vi "ConfigureMcsaAcquisition.vi"(8 "error in (no error)":errorcluster) -> (0 "error out":errorcluster, 2 "register data sets":T1[](array[typedef]), 3 "Mcsa Acquisition Config":T4 {"FixedSizeX31"."InputConfig" items=["AC Coupled", "DC Coupled", "IEPE AC Coupled"]}, 5 "valid":bool)   [LabVIEW 2017, in "McsaFpgaAcquisition.lvlib"]
uses:
  <vilib>/addons/InsightCM/Devices/Shared/Mcsa/McsaFpgaAcquisition/McsaFpgaAcquisition.lvlib
  <vilib>/addons/InsightCM/Devices/Shared/Mcsa/McsaFpgaAcquisition/controls/Configuration.ctl
  <vilib>/addons/InsightCM/Devices/Shared/Cms/CmsAcquisition/controls/FixedSizeArrays.ctl
  <vilib>/LabVIEW Targets/FPGA/cRIO/shared/nicrio_ModuleControls/nicrio_cRIO-9232_ConfigModeRing.ctl
  <vilib>/addons/InsightCM/Devices/Shared/Cms/cRIOWfmAcq/subVIs/RIO Wfm Cust Ctrls/rwfm_SamplingInfo.ctl
  <vilib>/addons/InsightCM/Devices/Shared/Mcsa/McsaFpgaAcquisition/controls/Group.ctl
  <vilib>/addons/InsightCM/Devices/Shared/Mcsa/McsaFpgaAcquisition/controls/ChannelMcsa.ctl
  <vilib>/addons/InsightCM/Devices/Shared/Mcsa/McsaFpgaAcquisition/controls/RangeParams.ctl
  <vilib>/addons/InsightCM/Devices/Shared/Mcsa/McsaDataEventCreator/controls/RegisterDataSets.ctl
  <vilib>/addons/InsightCM/Devices/Shared/Mcsa/McsaDataEventCreator/controls/Registry_DataSet.ctl
  <vilib>/addons/InsightCM/Devices/Shared/Mcsa/McsaDataEventCreator/controls/DataSetType.ctl
  <vilib>/addons/InsightCM/Utilities/GlobalConfiguration/GlobalConfiguration.lvlib
  <vilib>/addons/InsightCM/Devices/Shared/Cms/cRIOWfmAcq/cRIOWfmLib.lvlib
  <vilib>/addons/InsightCM/Devices/Shared/Cms/CmsAcquisition/CmsAcquisition.lvlib
  <vilib>/addons/InsightCM/Devices/Shared/Mcsa/McsaDataEventCreator/McsaDataEventCreator.lvlib
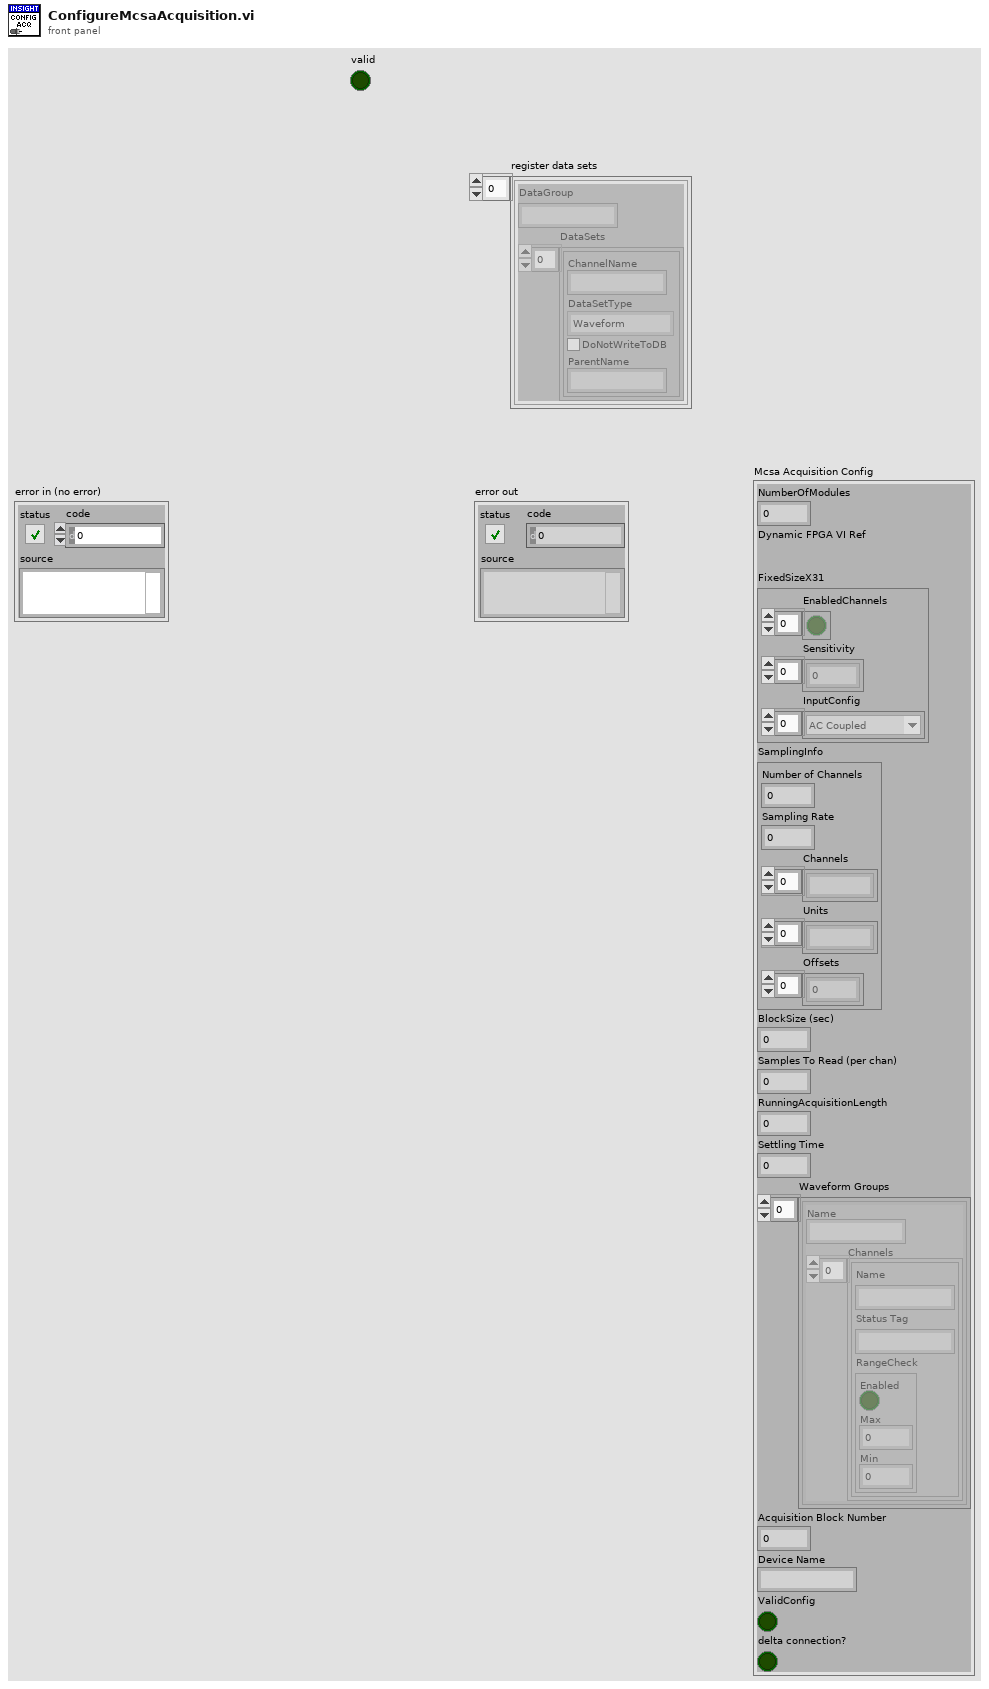
[diagram p1: front panel]
types:
  T1 = typedef "McsaDataEventCreator.lvlib/RegisterDataSets.ctl" = cluster{"DataGroup":string, "DataSets":T2[]}
  T2 = typedef "McsaDataEventCreator.lvlib/Registry_DataSet.ctl" = cluster{"ChannelName":string, "DataSetType":T3, "DoNotWriteToDB":bool, "ParentName":string}
  T3 = typedef "McsaDataEventCreator.lvlib/DataSetType.ctl" = enum16{"Waveform", "MCSAFFT", "TorqueWFM"}
  T4 = typedef "McsaFpgaAcquisition.lvlib/Configuration.ctl" = cluster{"NumberOfModules":i16, "Dynamic FPGA VI Ref":refnum<k20>, "FixedSizeX31":T5, "SamplingInfo":T7, "BlockSize (sec)":dbl, "Samples To Read (per chan)":i32, "RunningAcquisitionLength":dbl, "Settling Time":dbl, "Waveform Groups":T8[], "Acquisition Block Number":i32, "Device Name":string, "ValidConfig":bool, "delta connection?":bool}
  T5 = typedef "CmsAcquisition.lvlib/FixedSizeArrays.ctl" = cluster{"EnabledChannels":bool[], "Sensitivity":dbl[], "InputConfig":T6[]}
  T6 = typedef "nicrio_cRIO-9232_ConfigModeRing.ctl" = u8
  T7 = typedef "cRIOWfmLib.lvlib/rwfm_SamplingInfo.ctl" = cluster{"Number of Channels":i32, "Sampling Rate":dbl, "Channels":string[], "Units":string[], "Offsets":sgl[]}
  T8 = typedef "McsaFpgaAcquisition.lvlib/Group.ctl" = cluster{"Name":string, "Channels":T9[]}
  T9 = typedef "McsaFpgaAcquisition.lvlib/ChannelMcsa.ctl" = cluster{"Name":string, "Status Tag":string, "RangeCheck":T10}
  T10 = typedef "McsaFpgaAcquisition.lvlib/RangeParams.ctl" = cluster{"Enabled":bool, "Max":dbl, "Min":dbl}
  T11 = typedef "R2_Device.ctl" = cluster{"Id":string, "Name":string, "DeviceType":string, "HardwareName":string, "IpAddress":string, "HardwareInfo":T12[], "ApplicationType":string, "ApplicationVersion":string, "EquipmentIds":string[], "ConfigurationVersion":string, "State":T13, "Properties":T12[], "DataGroups":T14[], "BurstModeTrigger":T18}
  T12 = typedef "KeyValuePair.ctl" = cluster{"Key":string, "Value":string}
  T13 = typedef "DeviceState.ctl" = cluster{"Disabled":bool}
  T14 = typedef "R2_DataGroup.ctl" = cluster{"Name":string, "OperatingStates":T15[], "Properties":T12[], "EquipmentIds":string[], "AssetNodeId":string}
  T15 = typedef "OperatingState.ctl" = cluster{"Name":string, "Properties":T12[], "Triggers":T16[]}
  T16 = typedef "Trigger.ctl" = cluster{"Type":string, "Expression":string, "Conditions":T17[]}
  T17 = typedef "Condition.ctl" = cluster{"Source":string, "Type":string, "Operator":string, "CompareTo":string, "DwellSeconds":dbl}
  T18 = typedef "BurstModeTrigger.ctl" = cluster{"Trigger":T16, "SampleRate":string, "AcquisitionLength":string}
  T19 = typedef "R2_Channel.ctl" = cluster{"Id":string, "DeviceId":string, "Name":string, "ChannelType":string, "HardwareKey":string, "HardwareChannel":string, "DataGroup":string, "Keywords":string[], "EquipmentIds":string[], "Properties":T12[], "Metrics":T20[], "AssetNodeId":string, "MeasType":string, "AssetName":string}
  T20 = typedef "Metric.ctl" = cluster{"Id":string, "Name":string, "Unit":string, "Properties":T12[], "MetricDefinitionInstanceId":string}
  T21 = typedef "SectionKeyValues.ctl" = cluster{"Section":string, "KeyValues":T12[]}
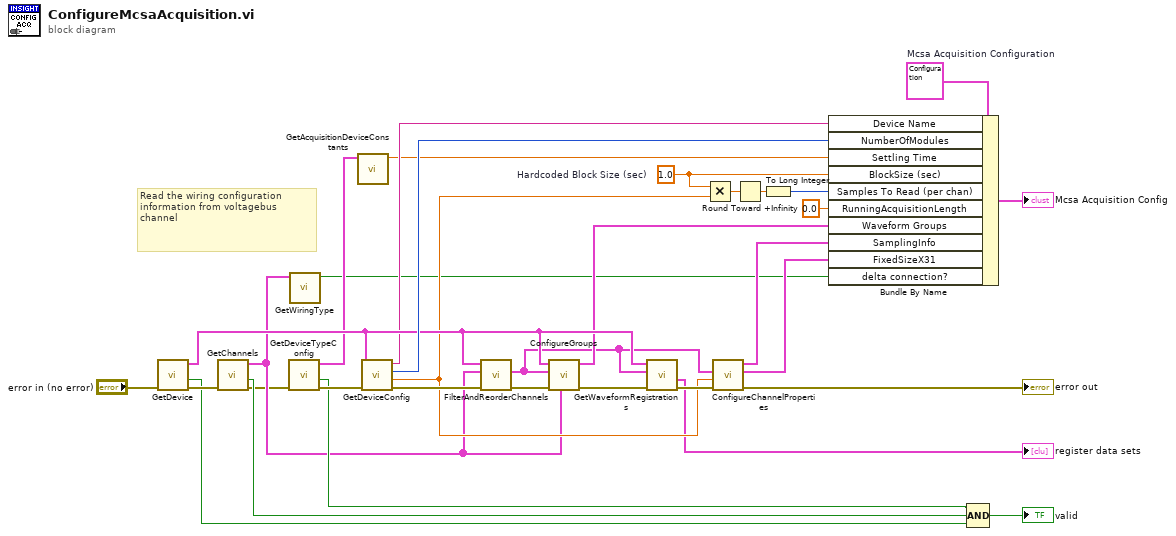
[diagram p0: block diagram]
diagram:
  w8 = T4 {"NumberOfModules"=0, "Dynamic FPGA VI Ref"=refnum, "FixedSizeX31"={"EnabledChannels"=[], "Sensitivity"=[], "InputConfig"=[]}, "SamplingInfo"={"Number of Channels"=0, "Sampling Rate"=0.0, "Channels"=[], "Units"=[], "Offsets"=[]}, "BlockSize (sec)"=0.0, "Samples To Read (per chan)"=0, "RunningAcquisitionLength"=0.0, "Settling Time"=0.0, "Waveform Groups"=[], "Acquisition Block Number"=0, "Device Name"="", "ValidConfig"=FALSE, "delta connection?"=FALSE}  # Mcsa Acquisition Configuration
  w29 = 1.0  # Hardcoded Block Size (sec)
  # "Read the wiring configuration information from voltagebus channel"
  n1 = call <vilib>:"GetDevice.vi"("error in (no error)"="error in (no error)") -> ("error out"=w32:errorcluster, "found"=w13:bool, "device configuration"=w18:T11)  [unwired: 8 in]
  n2 = call <vilib>:"GetChannels.vi"("error in (no error)"=w32) -> ("error out"=w1:errorcluster, "found"=w12:bool, "channels"=w3:T19[])  [unwired: 8 in]
  n3 = call <vilib>:"GetDeviceTypeConfig.vi"("error in (no error)"=w1) -> ("error out"=w10:errorcluster, "found"=w9:bool, "key values"=w6:T21[])  [unwired: 8 in]
  n4 = call <vilib>:"GetWiringType.vi"("channels"=w3) -> ("delta connection?"=w4:bool)  [unwired: 10 in]
  n5 = call <vilib>:"GetAcquisitionDeviceConstants.vi"("key values"=w6) -> ("settling time (seconds)"=w5:dbl)  [unwired: 10 in]
  n6 = call <vilib>:"GetDeviceConfig.vi"("error in (no error)"=w10, "Device"=w18) -> ("error out"=w23:errorcluster, "Sample Rate"=w7:dbl, "Number of Dynamic Modules"=w26:i32, "Name"=w15:string)  [unwired: 6 in]
  n7 = call <vilib>:"FilterAndReorderChannels.vi"("error in (no error)"=w23, "channels"=w3, "device"=w18) -> ("error out"=w21:errorcluster, "acquisition channels (in acquisition order)"=w14:T19[])  [unwired: 7 in]
  n8 = call <vilib>:"ConfigureGroups.vi"("all channels"=w3, "error in (no error)"=w21, "acquisition channels (in acquisition order)"=w14, "device"=w18) -> ("error out"=w20:errorcluster, "groups"=w16:T8[])  [unwired: 6 in]
  n9 = call <vilib>:"GetWaveformRegistrations.vi"("error in (no error)"=w20, "acquisition channels (in acquisition order)"=w14, "device"=w18) -> ("error out"=w19:errorcluster, "register data sets"=→"register data sets":T1[])  [unwired: 7 in]
  n10 = Multiply(x=w29, y=w7) -> (x*y=w31:dbl)
  n11 = call <vilib>:"ConfigureChannelProperties.vi"("error in (no error)"=w19, "Sampling Rate"=w7, "Filtered Channels (in acquisition order)"=w14) -> ("error out"=→"error out":errorcluster, "Channel Config X31"=w25:T5, "Sampling Info"=w17:T7)  [unwired: 6 in]
  n12 = Round Toward +Infinity(x=w31) -> (ceil(x): smallest int >= x=w30:dbl)
  n13 = To Long Integer(number=w30) -> (32bit integer=w28:i32)
  n14 = Bundle By Name(cluster=w8, "Device Name"=w15, "NumberOfModules"=w26, "Settling Time"=w5, "BlockSize (sec)"=w29, "Samples To Read (per chan)"=w28, "RunningAcquisitionLength"=0.0, "Waveform Groups"=w16, "SamplingInfo"=w17, "FixedSizeX31"=w25, "delta connection?"=w4) -> (→"Mcsa Acquisition Config":T4)
  n15 = Compound Arithmetic op=AND(w9, w12, w13) -> (→"valid":bool)
